vi "Configure Trend Wave.vi"(0 "VISA resource name":refnum<visa-resource-name>, 5 "Trend Direction (0 : Horizon)":i32(ring) items=["Horizon", "Vertical"], 7 "Enable Trend Clear On Start (False)":bool, 11 "error in (no error)":errorcluster) -> (4 "VISA resource name out":refnum<visa-resource-name>, 15 "error out":errorcluster)   [LabVIEW 2020, in "Yokogawa GX Series.lvlib"]
doc: "Sets the trend waveform display mode.\n\nCommand: STrdWave\n\nNote: This VI does nothing when the instrument is GM10."
uses:
  <instrlib>/Yokogawa GX Series/Yokogawa GX Series.lvlib
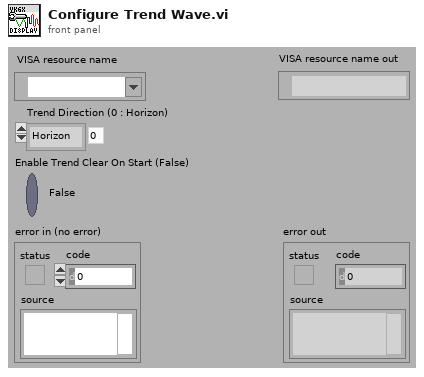
[diagram p1: front panel]
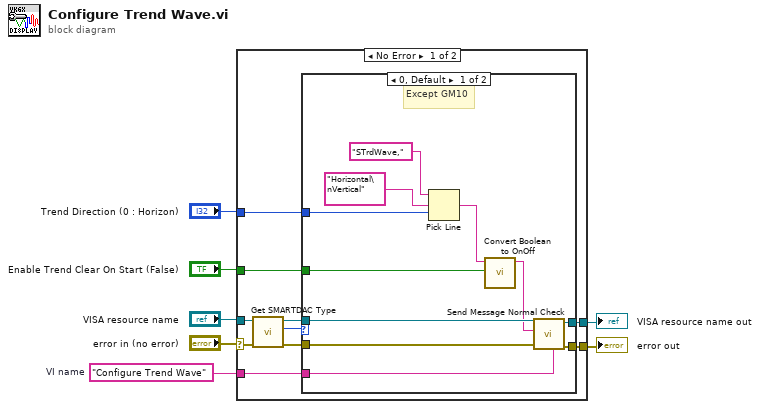
[diagram p0: block diagram]
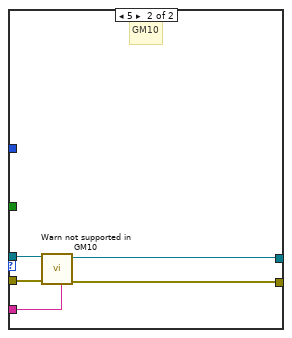
[diagram p2: hidden frame]
diagram:
  w4 = "Configure Trend Wave"  # VI name
  n1 = case shown="No Error" "error in (no error)" {
    selector: "error in (no error)" -> [w11 w34]
    tunnel: "Trend Direction (0 : Horizon)" -> [w17 _]
    tunnel: "VISA resource name" -> [w12 w35]
    tunnel: "Enable Trend Clear On Start (False)" -> [w16 _]
    tunnel: w4 -> [w15 _]
    tunnel: [w14 w35] -> w3
    tunnel: [w13 w34] -> w2
    frame No Error {
      n2 = call <instrlib>:"Get SMARTDAC Type.vi"("error in (no error)"=w11, "VISA resource name"=w12) -> ("error out"=w9:errorcluster, "SMARTDAC+ Type"=w8:u16, "VISA resource name out"=w10:refnum<visa-resource-name>)  [unwired: 7 in]
      n3 = case shown="0, Default" w8 {
        tunnel: w17 -> [w28 _]
        tunnel: w10 -> [w24 w33]
        tunnel: w16 -> [w22 _]
        tunnel: w15 -> [w21 w29]
        tunnel: [w20 w31] -> w14
        tunnel: [w19 w30] -> w13
        tunnel: w9 -> [w18 w32]
        frame 0, Default {
          # "Except GM10"
          n4 = Pick Line(string ("")="STrdWave," ("形式文字列"), multi-line string="Horizontal\nVertical", line index=w28) -> (output string=w25:string)
          n5 = call <instrlib>:"Convert Boolean to OnOff.vi"("On/Off"=w22, "Initial String (\"\")"=w25) -> ("Resulting String"=w23:string)  [unwired: 9 in]
          n6 = call <instrlib>:"Send Message Normal Check.vi"("Source (\"\")"=w21, "error in (no error)"=w18, "Send Message (\"\")"=w23, "VISA resource name"=w24) -> ("error out"=w19:errorcluster, "VISA resource name out"=w20:refnum<visa-resource-name>)  [unwired: 2 in, 4 out]
        }
        frame 5 {
          # "GM10"
          n7 = call <instrlib>:"Warn not supported in GM10.vi"("Source (\"\")"=w29, "error in (no error)"=w32, "VISA resource name"=w33) -> ("error out"=w30:errorcluster, "VISA resource name out"=w31:refnum<visa-resource-name>)  [unwired: 7 in]
        }
      }
    }
    frame Error {
    }
  }
  "error out" <- w2
  "VISA resource name out" <- w3
